vi "Execution Unit.Async.vi"(10 "Parameters":variant, 11 "Process":refnum<class "Process.lvclass">) -> ()   [LabVIEW 2023, in "Ballard MIL-STD-1553 Engine Support.lvlib" / "Custom Device.lvlib"]
uses:
  Custom Device.lvlib
  <vilib>/NI/NIVS Inline Async API/_VS Inline Async API/Process/Process.lvclass
  <vilib>/NI/NIVS Inline Async API/_Data Access Engine/Data Access Engine/Data Access Engine.lvclass
  Asynchronous Execution Unit Runtime Information.ctl
  Interfaces/Execution Unit/Execution Unit.lvclass
  Interfaces/Shared Resources/Shared Resources.lvclass
  Asynchronous Process Parameters.ctl
  <vilib>/NI/NIVS Inline Async API/_Data Access Engine/Access Type Classes/ReadWrite/ReadWrite.lvclass
  <vilib>/NI/NIVS Inline Async API/_Data Access Engine/Data Access Engine/Methods/Read.Lookup.vi
  <vilib>/NI/NIVS Inline Async API/_Data Access Engine/Data Access Engine/Methods/ReadWrite.Lookup.vi
  <vilib>/NI/NIVS Inline Async API/_Data Access Engine/Data Access Engine/Methods/Write.Lookup.vi
  <vilib>/NI/NIVS Inline Async API/_Data Access Engine/Data Access Engine/Methods/ReadWrite.Data.vi
  <vilib>/NI/NIVS Inline Async API/_Data Access Engine/Data Access Engine/Methods/Read.Data.vi
  <vilib>/NI/NIVS Inline Async API/_Data Access Engine/Data Access Engine/Methods/Write.Data.vi
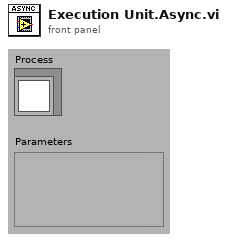
[diagram p1: front panel]
types:
  T1 = typedef "Ballard MIL-STD-1553 Engine Support.lvlib/Custom Device.lvlib/Asynchronous Process Parameters.ctl" = cluster{"Grouped Asynchronous Execution Unit Runtime Information":T2[], "shared resources":refnum<class "Shared Resources.lvclass">}
  T2 = typedef "Ballard MIL-STD-1553 Engine Support.lvlib/Custom Device.lvlib/Asynchronous Execution Unit Runtime Information.ctl" = cluster{"Execution Unit":refnum<class "Execution Unit.lvclass">, "Incoming Channel Group Name":string, "Outgoing Channel Group Name":string, "ReadWrite Channel Group Name":string}
  T3 = typedef "Data Access Engine.lvlib/Data Access Engine.lvclass/Write.DVR.ctl" = refnum<data-value>
  T4 = typedef "Data Access Engine.lvlib/Data Access Engine.lvclass/ReadWrite.DVR.ctl" = refnum<data-value>
  T5 = typedef "Data Access Engine.lvlib/Data Access Engine.lvclass/Read.DVR.ctl" = refnum<data-value>
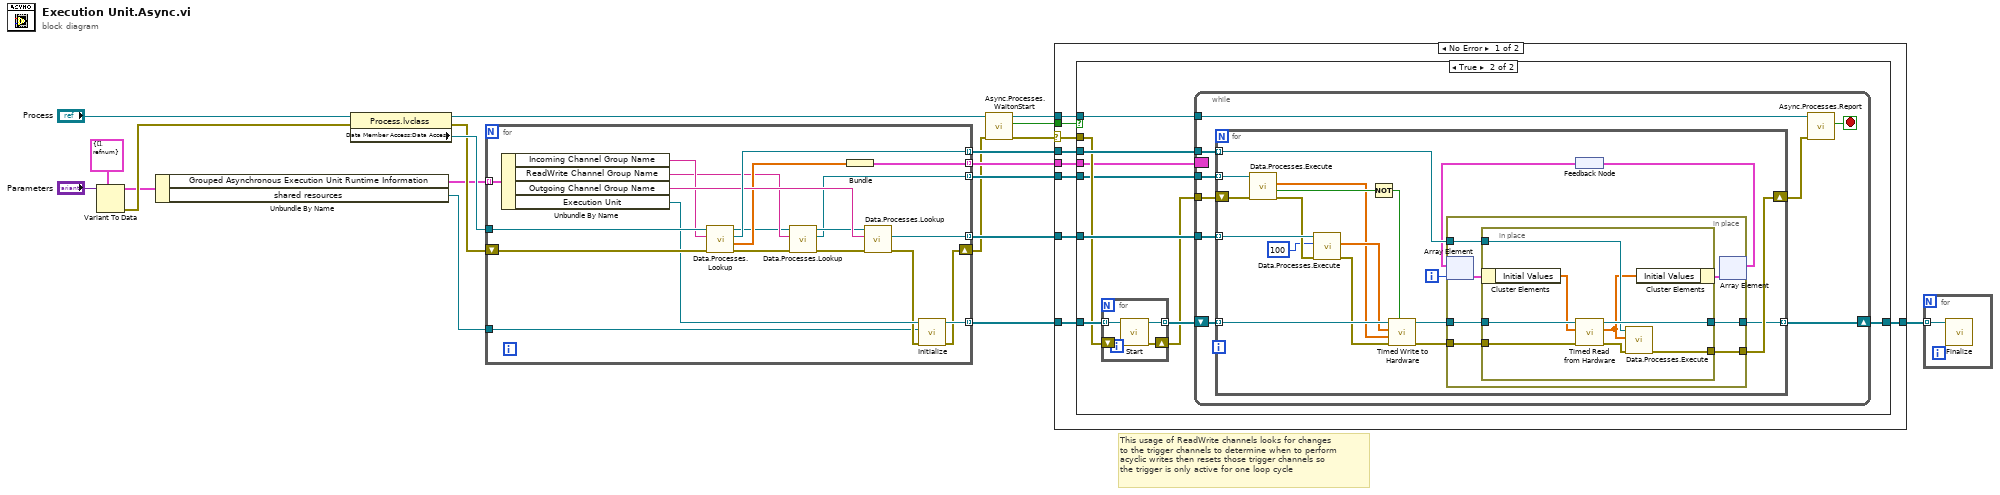
[diagram p0: block diagram]
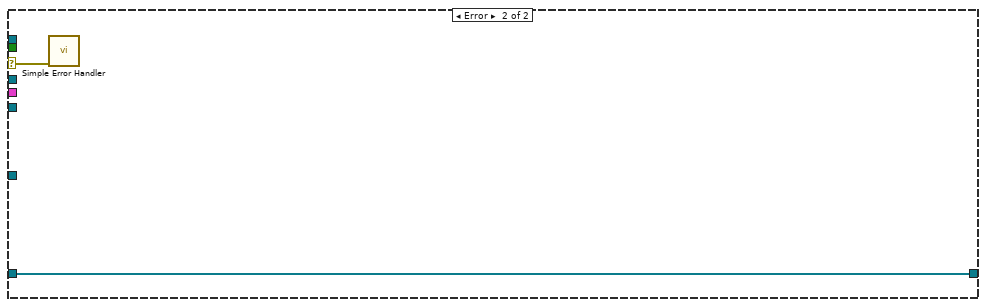
[diagram p3: hidden frame]
diagram:
  # "This usage of ReadWrite channels looks for changes\nto the trigger channels to determine when to perform\nacyclic writes then resets those trigger channels so\nthe trigger is only active for one loop cycle"
  n1 = Variant To Data(type=T1 {"Grouped Asynchronous Execution Unit Runtime Information"=[], "shared resources"=refnum} ("Asynchronous Process Parameters"), Variant="Parameters") -> (data=w8:T1, error out=w9:errorcluster)  [unwired: 1 in]
  n2 = Unbundle By Name(w8) -> ("Grouped Asynchronous Execution Unit Runtime Information"=w1:T2[], "shared resources"=w3:refnum<class "Shared Resources.lvclass">)
  n3 = property class="Process.lvclass"(reference="Process", error in=w9) -> (reference out=w14:refnum<class "Process.lvclass">, error out=w12:errorcluster, "Data Member Access:Data Access"=w13:refnum<class "Data Access Engine.lvclass">)
  n4 = for {
    tunnel: [w40] -> w17 mode=indexing
    tunnel: [w39] -> w16 mode=indexing
    tunnel: w13 -> [w38]
    tunnel: [w21] -> w7 mode=indexing
    tunnel: [w33] -> w6 mode=indexing
    tunnel: [w26] -> w4 mode=indexing
    tunnel: w3 -> [w23]
    shift-right: [w31] -> w2
    shift-left: w12 -> [w37]
    tunnel: w1 -> [w22] mode=indexing
    n5 = Unbundle By Name(w22) -> ("Incoming Channel Group Name"=w30:string, "ReadWrite Channel Group Name"=w29:string, "Outgoing Channel Group Name"=w36:string, "Execution Unit"=w34:refnum<class "Execution Unit.lvclass">)
    n6 = call-poly <vilib>:"Data.Processes.Lookup.vi"("error in (no error)"=w37, "Name"=w30, "Data Access API in"=w38) -> ("error out"=w25:errorcluster, "Initial Values"=w35:dbl[], "Ref"=w39:T3, "Data Access API out"=w28:refnum<class "Data Access Engine.lvclass">)  [unwired: 5 in]
    n7 = call-poly <vilib>:"Data.Processes.Lookup.vi"("error in (no error)"=w25, "Name"=w29, "Data Access API in"=w28) -> ("error out"=w24:errorcluster, "Ref"=w26:T4, "Data Access API out"=w27:refnum<class "Data Access Engine.lvclass">)  [unwired: 5 in, 1 out]
    n8 = Bundle("Initial Values"=w35) -> (w21:cluster{"Initial Values":dbl[]})  [unwired: 1 in]
    n9 = call-poly <vilib>:"Data.Processes.Lookup.vi"("error in (no error)"=w24, "Name"=w36, "Data Access API in"=w27) -> ("error out"=w32:errorcluster, "Ref"=w40:T5)  [unwired: 5 in, 2 out]
    n10 = call-dynamic "Initialize.vi"("error in (no error)"=w32, "shared resources"=w23, "Execution Unit in"=w34) -> ("error out"=w31:errorcluster, "Execution Unit out"=w33:refnum<class "Execution Unit.lvclass">)  [unwired: 7 in]
  }
  n11 = call <vilib>:"Async.Processes.WaitonStart.vi"("error in (no error)"=w2, "Process"=w14) -> ("error out"=w18:errorcluster, "Execute"=w20:bool, "Process out"=w19:refnum<class "Process.lvclass">)  [unwired: 7 in]
  n12 = case shown="No Error" w18 {
    selector: w18 -> [w45 w109]
    tunnel: w20 -> [w49 _]
    tunnel: w19 -> [w48 _]
    tunnel: w16 -> [w47 _]
    tunnel: w17 -> [w46 _]
    tunnel: w7 -> [w44 _]
    tunnel: w6 -> [w43 w108]
    tunnel: [w42 w108] -> w5
    tunnel: w4 -> [w41 _]
    frame No Error {
      n13 = case shown="True" w49 {
        tunnel: w45 -> [_ w56]
        tunnel: w48 -> [_ w58]
        tunnel: w46 -> [_ w60]
        tunnel: w47 -> [_ w59]
        tunnel: w44 -> [_ w54]
        tunnel: w43 -> [w50 w57]
        tunnel: [w50 w53] -> w42
        tunnel: w41 -> [_ w52]
        frame False {
        }
        frame True {
          n14 = for {
            tunnel: w57 -> [w64] mode=indexing
            tunnel: [w62] -> w55 mode=indexing
            shift-right: [w61] -> w51
            shift-left: w56 -> [w63]
            n15 = call-dynamic "Start.vi"("error in (no error)"=w63, "Execution Unit in"=w64) -> ("error out"=w61:errorcluster, "Execution Unit out"=w62:refnum<class "Execution Unit.lvclass">)  [unwired: 8 in]
          }
          n16 = while {
            tunnel: w58 -> [w73]
            tunnel: w60 -> [w71]
            tunnel: w59 -> [w70]
            border: w54 -> [_]
            shift-right: [w67] -> w53
            shift-left: w55 -> [w69]
            tunnel: w52 -> [w66]
            tunnel: w51 -> [w65]
            stop <- w72 stop-if-true
            n17 = for {
              tunnel: w71 -> [w92] mode=indexing
              tunnel: w70 -> [w91] mode=indexing
              tunnel: w69 -> [w90] mode=indexing
              tunnel: [w86] -> w67 mode=indexing
              tunnel: w66 -> [w85] mode=indexing
              shift-right: [w87] -> w68
              shift-left: w65 -> [w84]
              i -> [w79]
              n18 = call-poly <vilib>:"Data.Processes.Execute.vi"("error in (no error)"=w84, "Ref"=w85) -> ("error out"=w83:errorcluster, "Timeout?"=w81:bool, "Data"=w74:dbl[])  [unwired: 6 in, 1 out]
              n19 = call-poly <vilib>:"Data.Processes.Execute.vi"("error in (no error)"=w83, "timeout ms"=100, "Ref"=w92) -> ("error out"=w88:errorcluster, "Values"=w75:dbl[])  [unwired: 6 in, 1 out]
              n20 = Not(x=w81) -> (.not. x?=w76:bool)
              n21 = call "Timed Write to Hardware.vi"("Triggers Valid"=w76, "error in"=w88, "Trigger Values"=w74, "Values"=w75, "Execution Unit in"=w90) -> ("error out"=w82:errorcluster, "Execution Unit out"=w89:refnum<class "Execution Unit.lvclass">)  [unwired: 3 in, 2 out]
              n22 = feedback #1() -> (w78:cluster{"Initial Values":dbl[]}[])
              n23 = in-place {
                in-place-border: w91 -> [w99]
                in-place-border: w89 -> [w98]
                in-place-border: [w97] -> w87
                in-place-border: [w96] -> w86
                in-place-border: w82 -> [w95]
                n24 = in-place-array #2(w78, w79) -> (w94:cluster{"Initial Values":dbl[]})
                n25 = in-place {
                  in-place-border: w99 -> [w102]
                  in-place-border: w98 -> [w107]
                  in-place-border: [w105] -> w97
                  in-place-border: [w104] -> w96
                  in-place-border: w95 -> [w103]
                  n26 = in-place-cluster #3(w94) -> ("Initial Values"=w101:dbl[])
                  n27 = call "Timed Read from Hardware.vi"("error in"=w103, "Values in"=w101, "Execution Unit in"=w107) -> ("error out"=w106:errorcluster, "Values out"=w100:dbl[], "Execution Unit out"=w104:refnum<class "Execution Unit.lvclass">)  [unwired: 6 in]
                  n28 = call-poly <vilib>:"Data.Processes.Execute.vi"("error in (no error)"=w106, "Values"=w100, "Ref"=w102) -> ("error out"=w105:errorcluster)  [unwired: 8 in]
                  n29 = in-place-cluster #3("Initial Values"=w100) -> (w93:cluster{"Initial Values":dbl[]})
                }
                n30 = in-place-array #2(w93) -> (w77:cluster{"Initial Values":dbl[]}[])  [unwired: 1 out]
              }
              n31 = feedback-in #1(w77) -> ()
            }
            n32 = call <vilib>:"Async.Processes.Report.vi"("Error"=w68, "Process in"=w73) -> ("Stop"=w72:bool)  [unwired: 8 in, 1 out]
          }
        }
      }
    }
    frame Error {
      n33 = call <vilib>:"Simple Error Handler.vi"("error in (no error)"=w109) -> ()  [unwired: 4 in, 5 out]
    }
  }
  n34 = for {
    tunnel: w5 -> [w110] mode=indexing
    n35 = call-dynamic "Finalize.vi"("Execution Unit in"=w110) -> ()  [unwired: 9 in, 2 out]
  }
